vi "First Step.vi"(8 "error in (no error)":errorcluster, 11 "Magnetic Field Lakeshore Scan.lvclass in":refnum<class "Magnetic Field Lakeshore Scan.lvclass">) -> (0 "error out":errorcluster, 2 "Current Position":dbl, 3 "Magnetic Field Lakeshore Scan.lvclass out":refnum<class "Magnetic Field Lakeshore Scan.lvclass">)   [LabVIEW 2023, in "Magnetic Field Lakeshore Scan.lvclass"]
doc: "(Dynamic) Reset the instrument and prepare to scan. Go to step #0 - the first step. If desired, the scanner may do this in a different way than usual (i.e. by preparing to move a long distance, or reset to home position.)"
uses:
  Magnetic Field Lakeshore Scan.lvclass
  Scanner/Scanner.lvclass
  Instruments/Utility Classes/Scannable/Scannable.lvclass
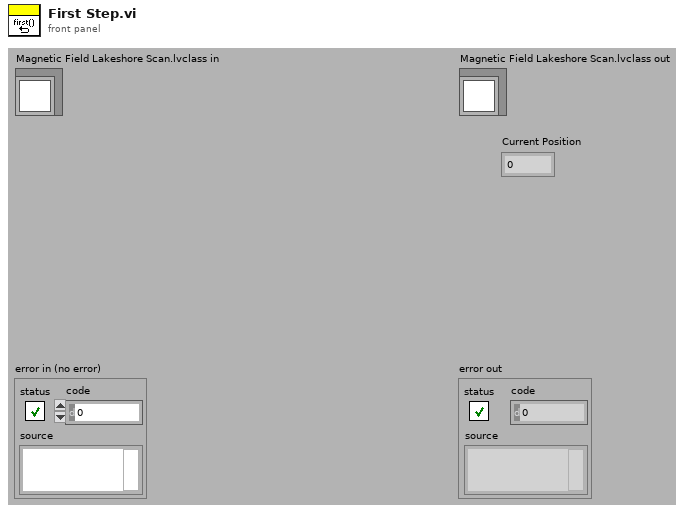
[diagram p1: front panel]
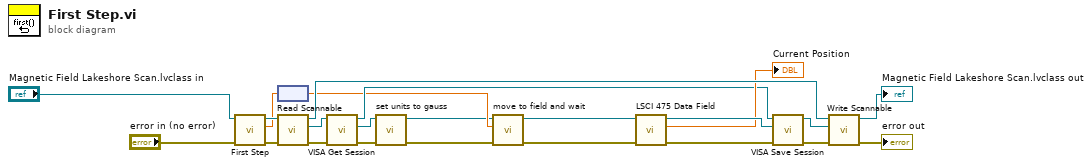
[diagram p0: block diagram]
diagram:
  n1 = call-parent "First Step.vi"("error in (no error)"="error in (no error)", "Scanner.lvclass in"="Magnetic Field Lakeshore Scan.lvclass in") -> ("error out"=w23:errorcluster, "Current Position"=w6:dbl, "Scanner.lvclass out"=w22:refnum<class "Magnetic Field Lakeshore Scan.lvclass">)  [unwired: 7 out]
  n2 = node(w6) -> (w5:dbl[unit])
  n3 = call-dynamic "Read Scannable.vi"("error in (no error)"=w23, "Scanner.lvclass in"=w22) -> ("error out"=w17:errorcluster, "Scannable.lvclass"=w8:refnum<class "Scannable.lvclass">, "Scanner.lvclass out"=w21:refnum<class "Magnetic Field Lakeshore Scan.lvclass">)  [unwired: 7 out]
  n4 = call-dynamic "VISA Get Session.vi"("error in (no error)"=w17, "Instrument.lvclass in"=w8) -> ("error out"=w2:errorcluster, "VISA Resource Name"=w4:refnum<visa-resource-name>, "Instrument.lvclass out"=w7:refnum<class "Scannable.lvclass">)  [unwired: 7 out]
  n5 = call "set units to gauss.vi"("VISA session"=w4, "error in (no error)"=w2) -> ("dup VISA session"=w3:refnum<visa-resource-name>, "error out"=w1:errorcluster)  [unwired: 7 in]
  n6 = call "move to field and wait.vi"("error in (no error)"=w1, "Setpoint"=w5, "VISA session"=w3) -> ("error out"=w12:errorcluster, "dup VISA session"=w14:refnum<visa-resource-name>)  [unwired: 7 in]
  n7 = call "LSCI 475 Data Field.vi"("error in (no error)"=w12, "VISA session"=w14) -> ("error out"=w11:errorcluster, "Field Reading"=→"Current Position":dbl, "dup VISA session"=w13:refnum<visa-resource-name>)  [unwired: 7 in]
  n8 = call-dynamic "VISA Save Session.vi"("error in (no error)"=w11, "VISA Resource Name"=w13, "Instrument.lvclass in"=w7) -> ("error out"=w16:errorcluster, "Instrument.lvclass out"=w15:refnum<class "Scannable.lvclass">)  [unwired: 7 out]
  n9 = call-dynamic "Write Scannable.vi"("error in (no error)"=w16, "Scannable.lvclass"=w15, "Scanner.lvclass in"=w21) -> ("error out"=→"error out":errorcluster, "Scanner.lvclass out"=→"Magnetic Field Lakeshore Scan.lvclass out":refnum<class "Magnetic Field Lakeshore Scan.lvclass">)  [unwired: 7 out]
